vi "AD（V3.1）.vi"(8 "N-length":dbl, 9 "M-length":dbl, 10 "hDevice":i32, 11 "pulDDR2Length":u32) -> (0 "幅频谱":dbl[](graph), 1 "时域谱":dbl[](graph), 3 "hDevice out":i32)   [LabVIEW 2016]
uses:
  <vilib>/Analysis/2dsp.llb/Real FFT.vi
  INF/amd64/PCI8502_32.dll
  <vilib>/Analysis/NI_AALPro.lvlib
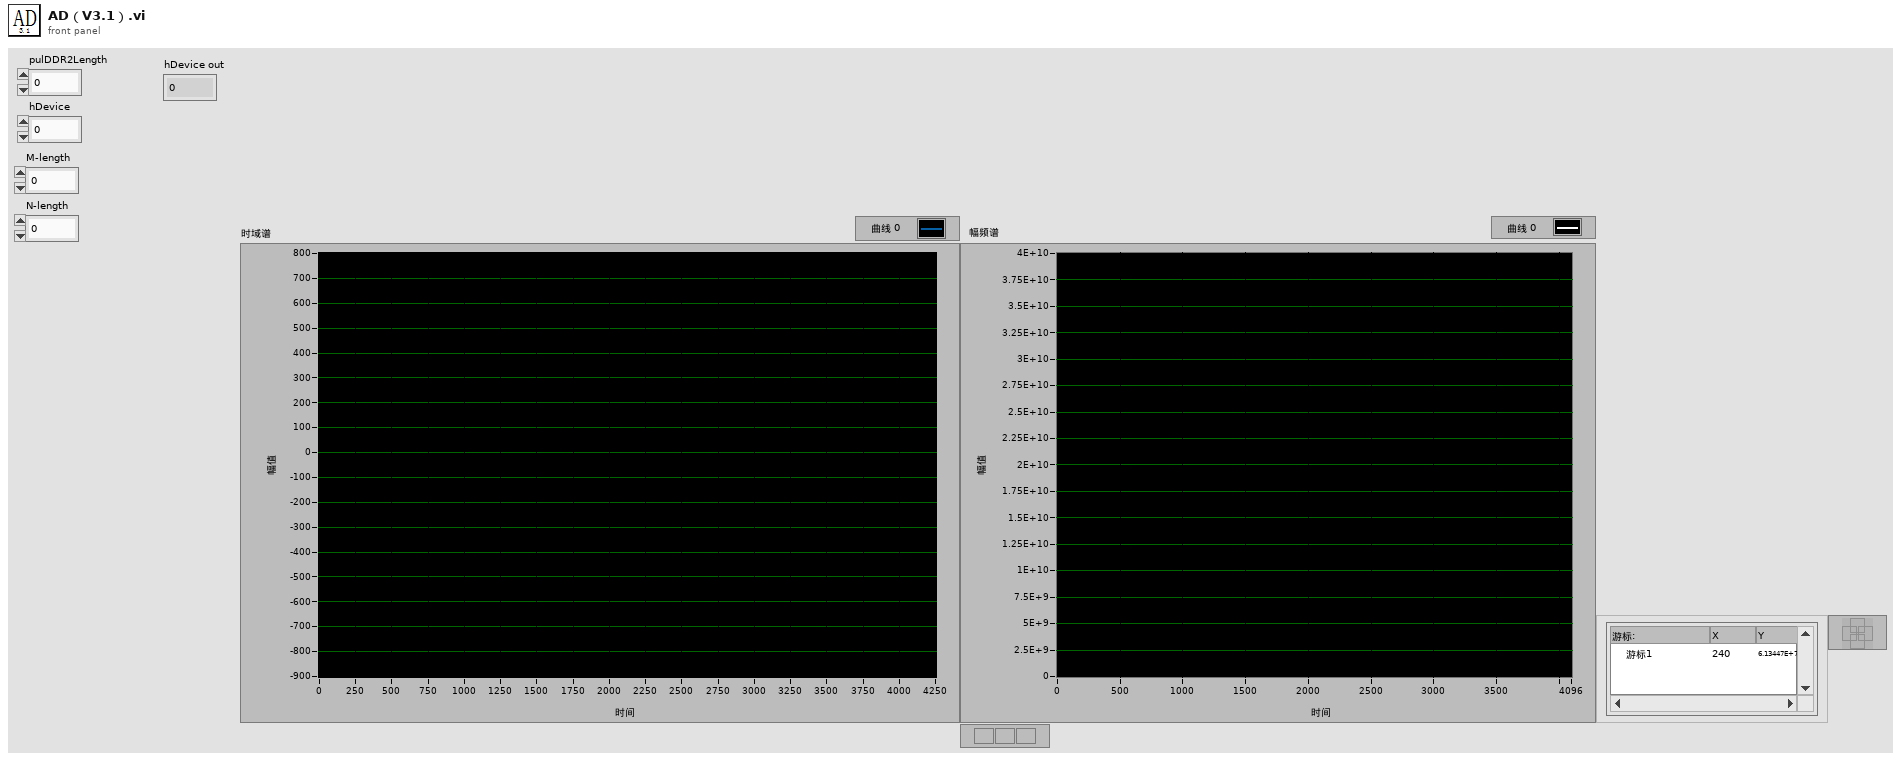
[diagram p1: front panel]
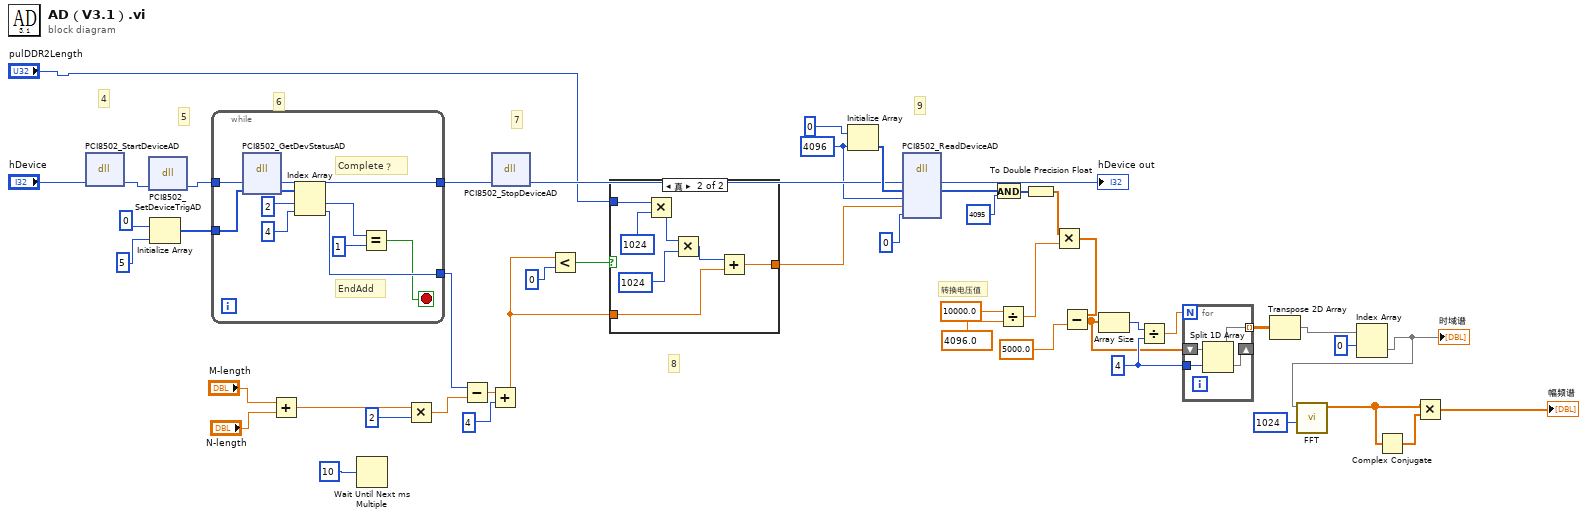
[diagram p0: block diagram]
diagram:
  w15 = 4
  w17 = 4096 ("dimension size")
  # "9"
  # "8"
  # "7"
  # "6"
  # "5"
  # "4"
  # "转换电压值"
  n1 = dll-call lib="PCI8502_32" fn="PCI8502_StartDeviceAD" label="StartDeviceAD"("hDevice"="hDevice") -> ("hDevice"=w47:i32)  [unwired: 4 in, 2 out]
  n2 = dll-call lib="PCI8502_32" fn="PCI8502_SetDeviceTrigAD" label="SetDeviceTrigAD"("hDevice"=w47) -> ("hDevice"=w24:i32)  [unwired: 4 in, 2 out]
  n3 = Initialize Array(0, 5) -> (w21:i32[])
  n4 = while {
    tunnel: [w53] -> w20
    tunnel: w24 -> [w52]
    tunnel: w21 -> [w51]
    tunnel: [w50] -> w18
    stop <- w49 stop-if-true
    # "EndAdd"
    # "Complete？"
    n5 = dll-call lib="PTH2aabs CUsersH301Desktopart闭环扫描程序采集卡控制INFamd64PCI8502_32.dll" fn="PCI8502_GetDevStatusAD" label="GetDevStatusAD"("hDevice"=w52, "pADStatus"=w51) -> ("hDevice"=w50:i32, "pADStatus"=w55:i32[])  [unwired: 4 in, 2 out]
    n6 = Index Array(array=w55, index #1=2, index #2=4) -> (element #1=w57:i32, element #2=w53:i32)
    n7 = Equal?(x=w57, y=1) -> (x = y?=w49:bool)
  }
  n8 = Add(x="M-length", y="N-length") -> (x+y=w19:dbl)
  n9 = Wait Until Next ms Multiple(millisecond multiple=u32 10) -> ()  [unwired: 1 out]
  n10 = Multiply(x=w19, y=u32 2) -> (x*y=w32:dbl)
  n11 = Subtract(x=w20, y=w32) -> (x-y=w34:dbl)
  n12 = Add(x=w34, y=u32 4) -> (x+y=w29:dbl)
  n13 = dll-call lib="PCI8502_32" fn="PCI8502_StopDeviceAD" label="StopDeviceAD"("hDevice"=w18) -> ("hDevice"=w35:i32)  [unwired: 4 in, 2 out]
  n14 = Less?(x=w29, y=u32 0) -> (x < y?=w25:bool)
  n15 = case shown="真" w25 {
    tunnel: w29 -> [w59 w62]
    tunnel: [w59 w61] -> w30
    tunnel: "pulDDR2Length" -> [_ w60]
    frame False {
    }
    frame True {
      n16 = Multiply(x=w60, y=u32 1024) -> (x*y=w65:u32)
      n17 = Multiply(x=w65, y=u32 1024) -> (x*y=w63:u32)
      n18 = Add(x=w63, y=w62) -> (x+y=w61:dbl)
    }
  }
  n19 = Initialize Array(0, w17) -> (w36:i32[])
  n20 = dll-call lib="PCI8502_32" fn="PCI8502_ReadDeviceAD" label="ReadDeviceAD"("hDevice"=w35, "ADBuffer"=w36, "nReadSizeWords"=w17, "ulStartAddr"=w30, "nRetSizeWords"=0) -> ("hDevice"=→"hDevice out":i32, "ADBuffer"=w27:u16[])  [unwired: 7 in, 2 out]
  n21 = And(x=w27, y=4095) -> (x .and. y?=w38:i32[])
  n22 = Divide(x=10000.0, y=4096.0) -> (x/y=w40:dbl)
  n23 = To Double Precision Float(number=w38) -> (double precision float=w41:dbl[])
  n24 = Multiply(x=w41, y=w40) -> (x*y=w39:dbl[])
  n25 = Subtract(x=w39, y=5000.0) -> (x-y=w13:dbl[])
  n26 = Array Size(array=w13) -> (size(s)=w16:i32)
  n27 = Divide(x=w16, y=w15) -> (x/y=w14:dbl)
  n28 = for {
    N: w14 -> [_]
    tunnel: w15 -> [w70]
    shift-right: [w68] -> _
    shift-left: w13 -> [w69]
    tunnel: [w67] -> w12 mode=indexing
    n29 = Split 1D Array(array=w69, index=w70) -> (first subarray=w67:dbl[], second subarray=w68:dbl[])
  }
  n30 = Transpose 2D Array(2D array=w12) -> (transposed array=w10:dbl[][])
  n31 = Index Array(array=w10, index (row)=0 ("索引 (行)")) -> (element=w8:dbl[])  [unwired: 1 in]
  "时域谱" <- w8
  n32 = call-poly <vilib>:"FFT.vi"("FFT size"=1024 ("m"), "X"=w8) -> ("FFT {X}"=w7:cdb[])  [unwired: 8 in, 1 out]
  n33 = Complex Conjugate(1:w7) -> (0:w6:cdb[])
  n34 = Multiply(x=w7, y=w6) -> (x*y=→"幅频谱":cdb[])
